vi "frontend.vi"() -> ()   [LabVIEW 2011]
uses:
  custom_modules/typedefs/point.ctl
  custom_modules/typedefs/control_cluster.ctl
  custom_modules/typedefs/preset_control_cluster.ctl
  custom_modules/typedefs/single_step_controls.ctl
  custom_modules/typedefs/camera_settings.ctl
  labview tests/states.ctl
  <vilib>/Utility/error.llb/DialogType.ctl
  stage_modules/Globals.vi
  <vilib>/vision/NI_Vision_Development_Module.lvlib
panel:
  in  "Single step controls":T1
  in  "emergency stop":bool
  in  "Control tabs":T2(tab)
  in  "File name base":string
  in  "Movement controls":T3={"Nx"=10, "Ny"=10, "X separation"=100, "Y separation"=100}
  in  "set origin button":bool
  in  "Preset controls":T4 {"Presets" items=["test1.preset", "test2.preset"]}
  in  "Origin":T5
  in  "PC connection port":u16(ring)=3 items=["PCI board", "COM 1", "TPL1", "COM3"]
  in  "close button":bool
  in  "Run test button":bool
  in  "params_changed":bool
  out "connection indicator":bool
  in  "stage adjusted":bool
  out "Most recent image":T6(plugin-control)
  out "Image index":i32
  out "Preview":T6(plugin-control)
  out "Histogram":T7(graph)
  in  "Camera settings":T8={"Gain"=1.0, "Exposure (s)"=0.05, "Preview binning"=2, "Capture binning"=0} {"Capture binning" items=["1x1", "2x2", "4x4", "8x8"]; "Preview binning" items=["1x1", "2x2", "4x4", "8x8"]; "Exposure (s)" scale=1e-05..1000.0 scale format="%^#_1e"; "Gain" scale=0.451..21.5 scale format="%#_3g"}
  in  "auto expose button":bool
  in  "Delay between captures (ms)":dbl=2000.0
  in  "Image Output directory":path=path "C:/Users/0800706m/Documents/microscope_software/output"
  in  "Preset directory":path=path "C:/Users/0800706m/Documents/microscope_software/presets"
  in  "Focal stack separation":dbl
  in  "Focal stack size":i32
  out "Array of positions":T5[](array[typedef])
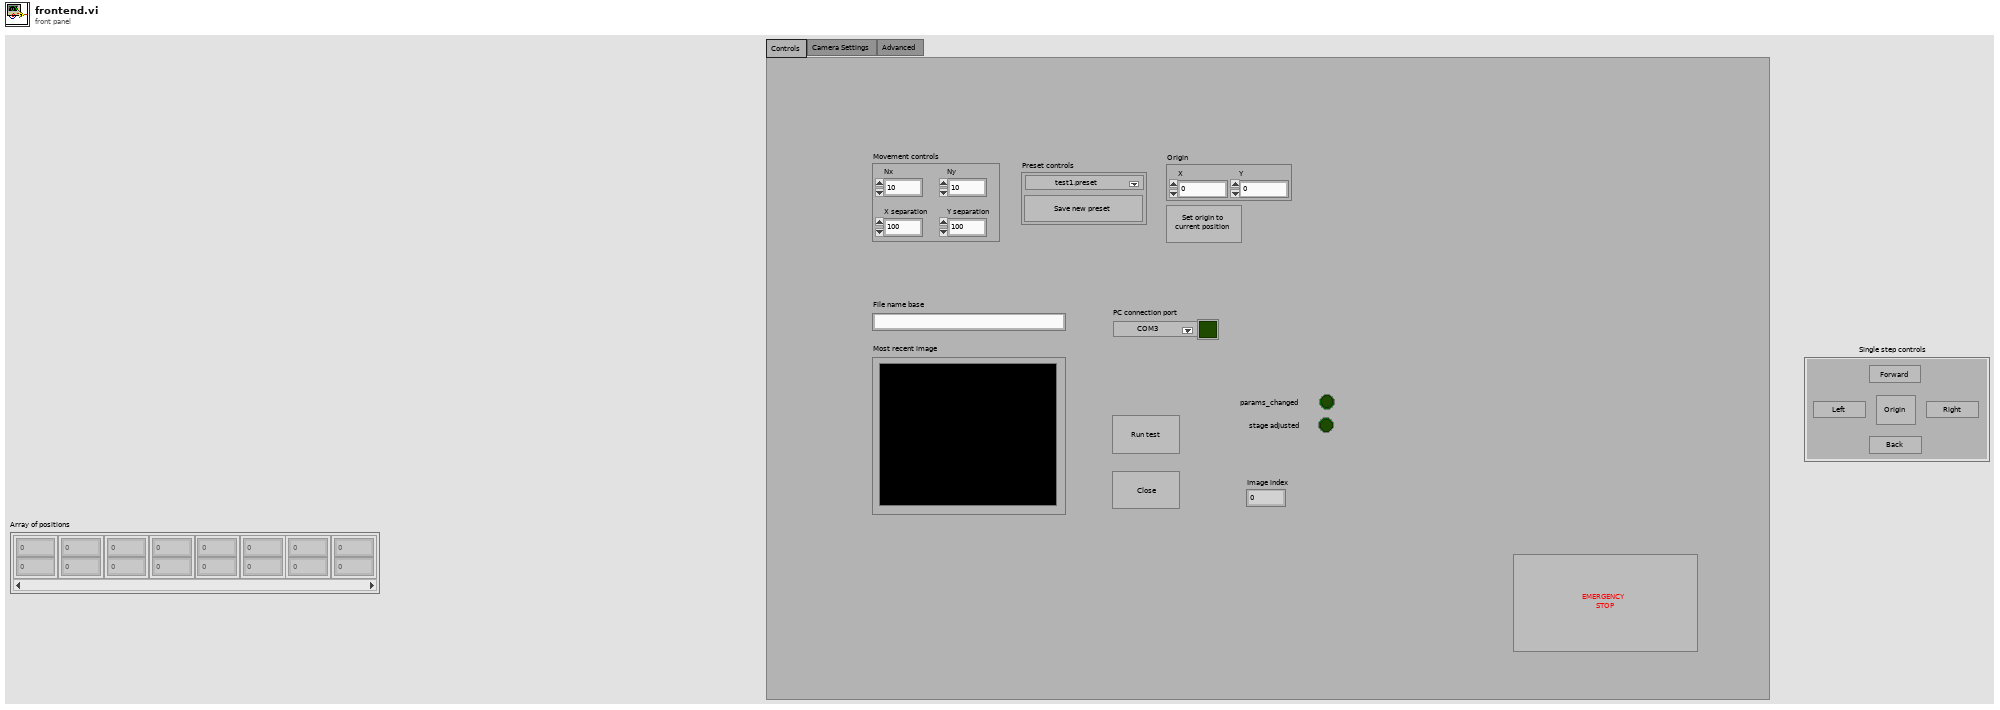
[diagram p1: front panel]
types:
  T1 = typedef "single_step_controls.ctl" = cluster{"move to origin button":bool, "Left":bool, "Right":bool, "Back":bool, "Forward":bool}
  T2 = enum32{"Controls", "Camera Settings", "Advanced"}
  T3 = typedef "control_cluster.ctl" = cluster{"Nx":i32, "Ny":i32, "X separation":i32, "Y separation":i32}
  T4 = typedef "preset_control_cluster.ctl" = cluster{"Presets":u16, "save preset button":bool}
  T5 = typedef "point.ctl" = cluster{"X":i32, "Y":i32}
  T6 = typedef "IMAQ Image.ctl" = refnum<image>
  T7 = cluster{"Starting Value":sgl, "Incremental Value":sgl, "Histogram":u32[]}
  T8 = typedef "camera_settings.ctl" = cluster{"Gain":dbl, "Exposure (s)":dbl, "Preview binning":u16, "Capture binning":u16}
  T9 = typedef "states.ctl" = enum16{"Init", "Check state", "Set parameters", "Preview", "Adjust stage", "Run test", "Close"}
  T10 = enum8{"Enabled", "Disabled", "Disabled and Grayed Out"}
  T11 = enum32{"gain", "offset", "exposure", "binning", "horizontal binning", "vertical binning", "readout speed", "trigger type", "lcd filter", "cooler", "exposure red", "exposure blue", "image format", "roi x", "roi y", "roi width", "roi height", "reserved1", "shutter state", "reserved2", "sync-b out", "reserved3", "intensifier gain", "trigger delay", "camera mode", "normalized gain", "normalized intenifier gain DB", "doPostProcessing", "postProcessGainRed", "postProcessGainGreen", "postProcessGainBlue", "postProcessBayerAlgorithm", "postProcessImageFormat", "fan", "blackout mode", "high sensitivity", "Readout Port", "EM Gain", "open delay", "close delay", "clearing mode"}
  T12 = typedef "Image Type" = u32
  T13 = cluster{"Refnum out":T6, "cameraId out":u32, "error out":errorcluster}
  T14 = cluster{"Global Rectangle":i32[], "Contours":cluster{"Contour Type":u32, "ROI Type":u32, "Points":i32[]}[]}
  T15 = cluster{"cameraId out":u32, "error out":errorcluster, "Image Out":T6}
  T16 = typedef "DialogType.ctl" = u16
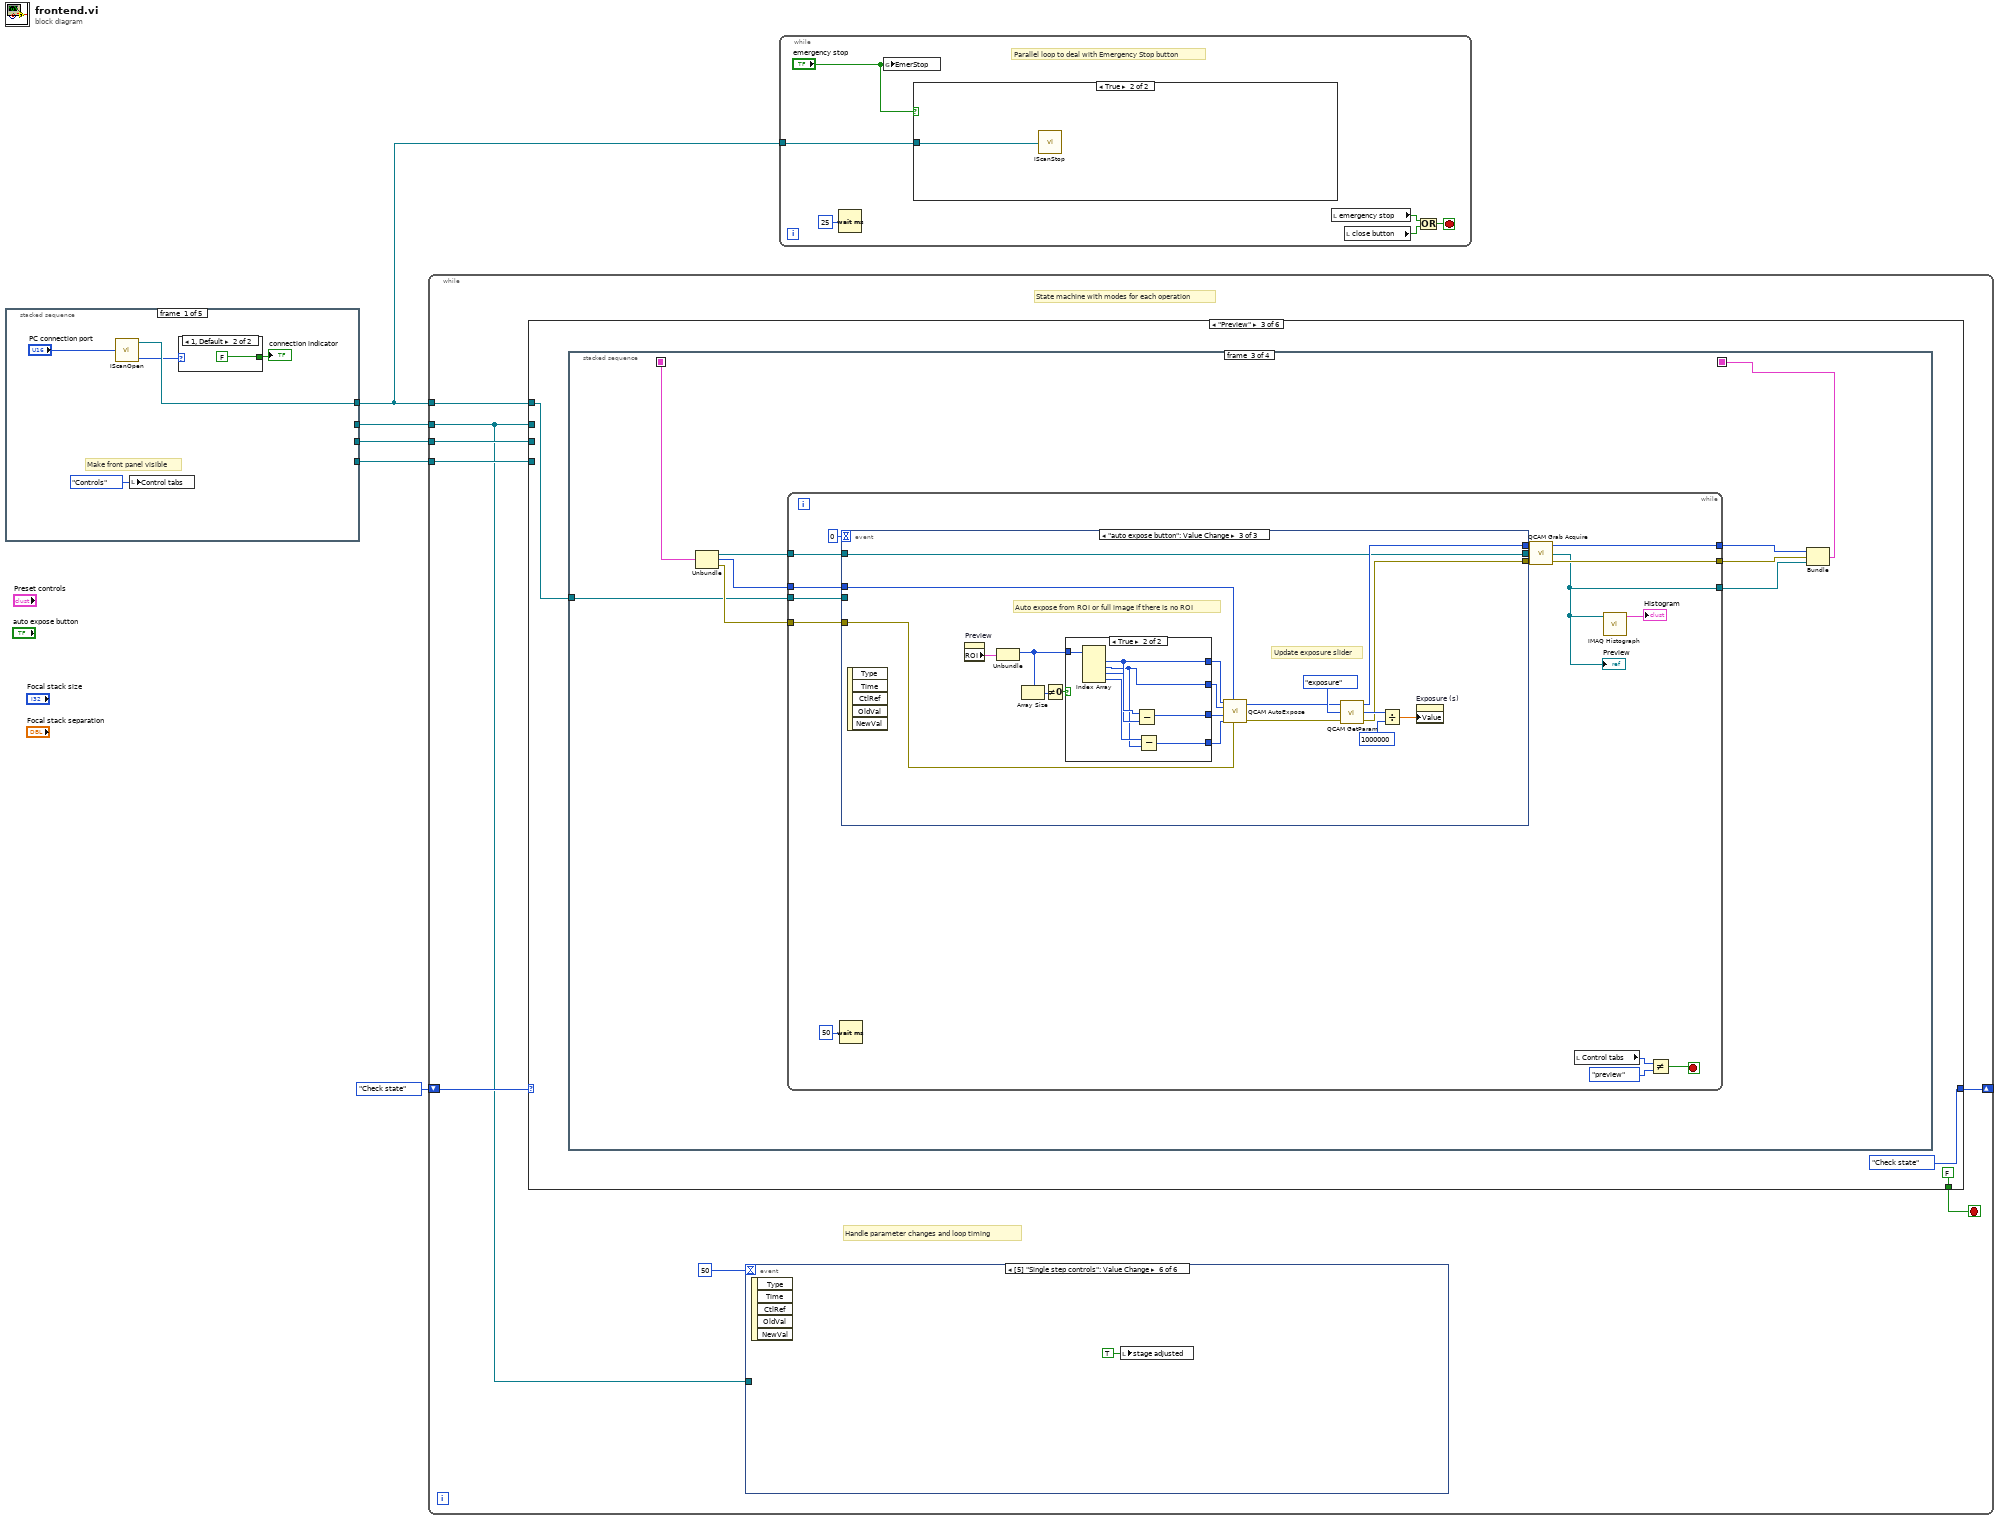
[diagram p0: block diagram]
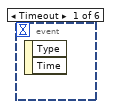
[diagram p3: hidden frame]
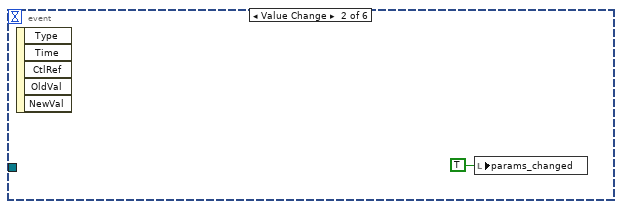
[diagram p4: hidden frame]
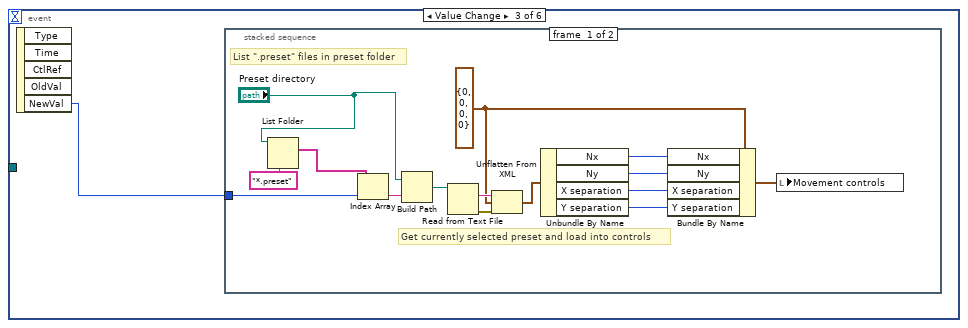
[diagram p5: hidden frame]
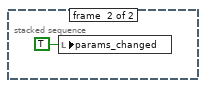
[diagram p6: hidden frame]
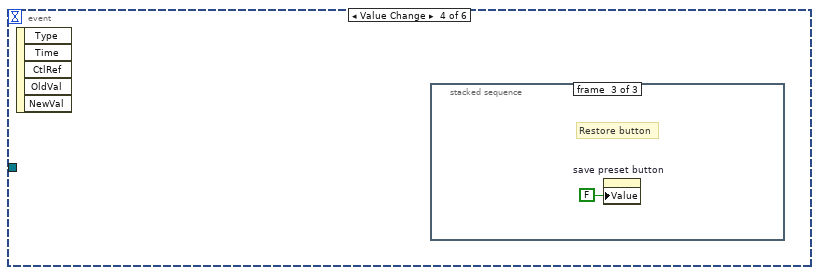
[diagram p7: hidden frame]
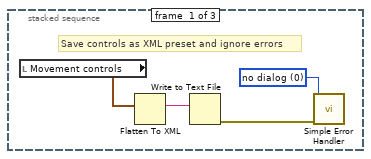
[diagram p8: hidden frame]
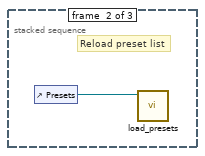
[diagram p9: hidden frame]
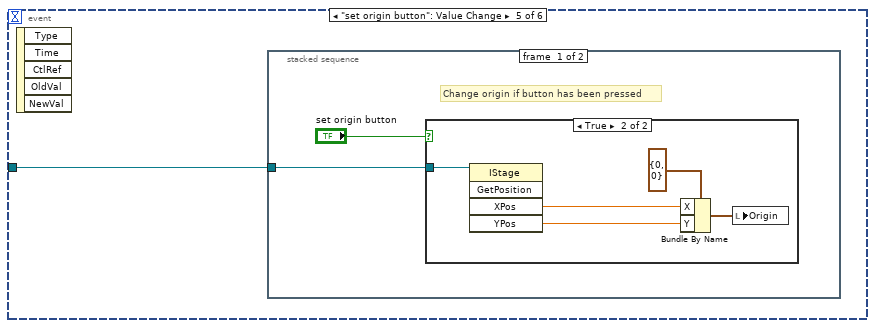
[diagram p10: hidden frame]
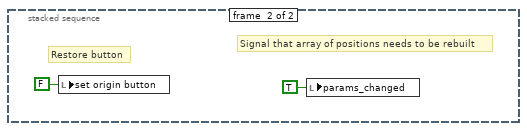
[diagram p12: hidden frame]
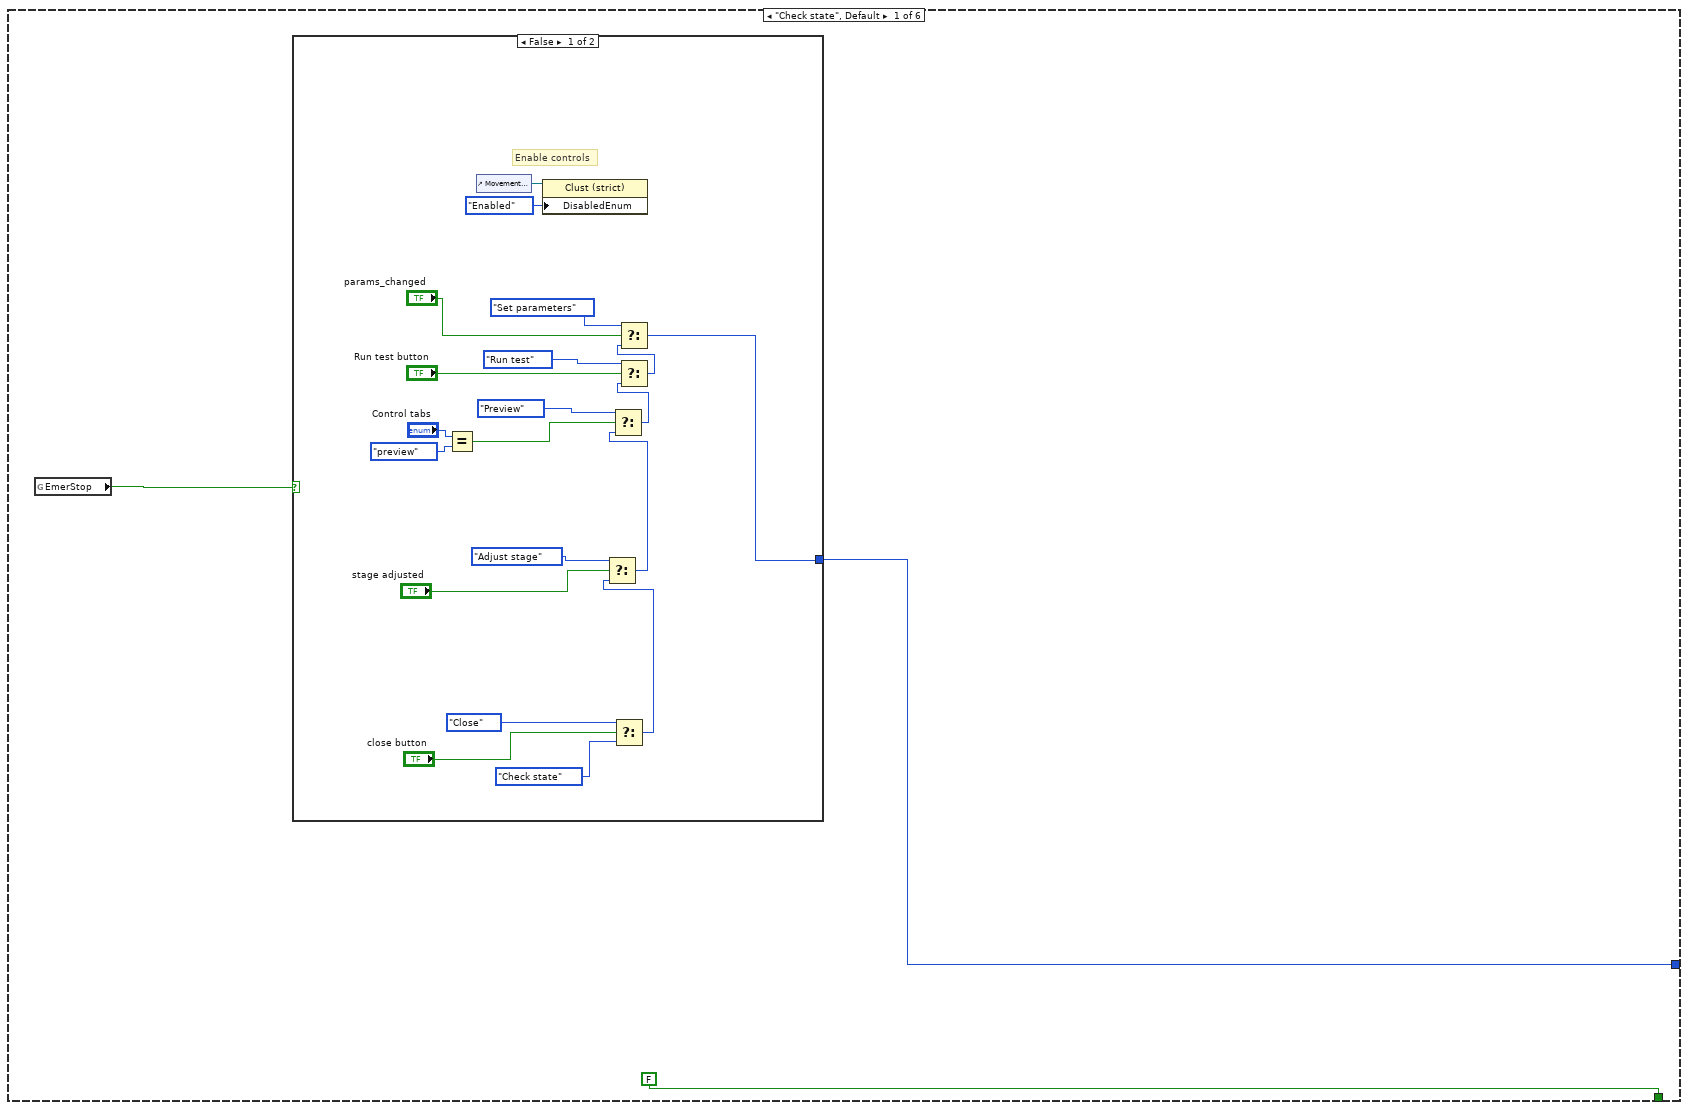
[diagram p13: hidden frame]
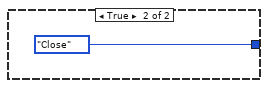
[diagram p14: hidden frame]
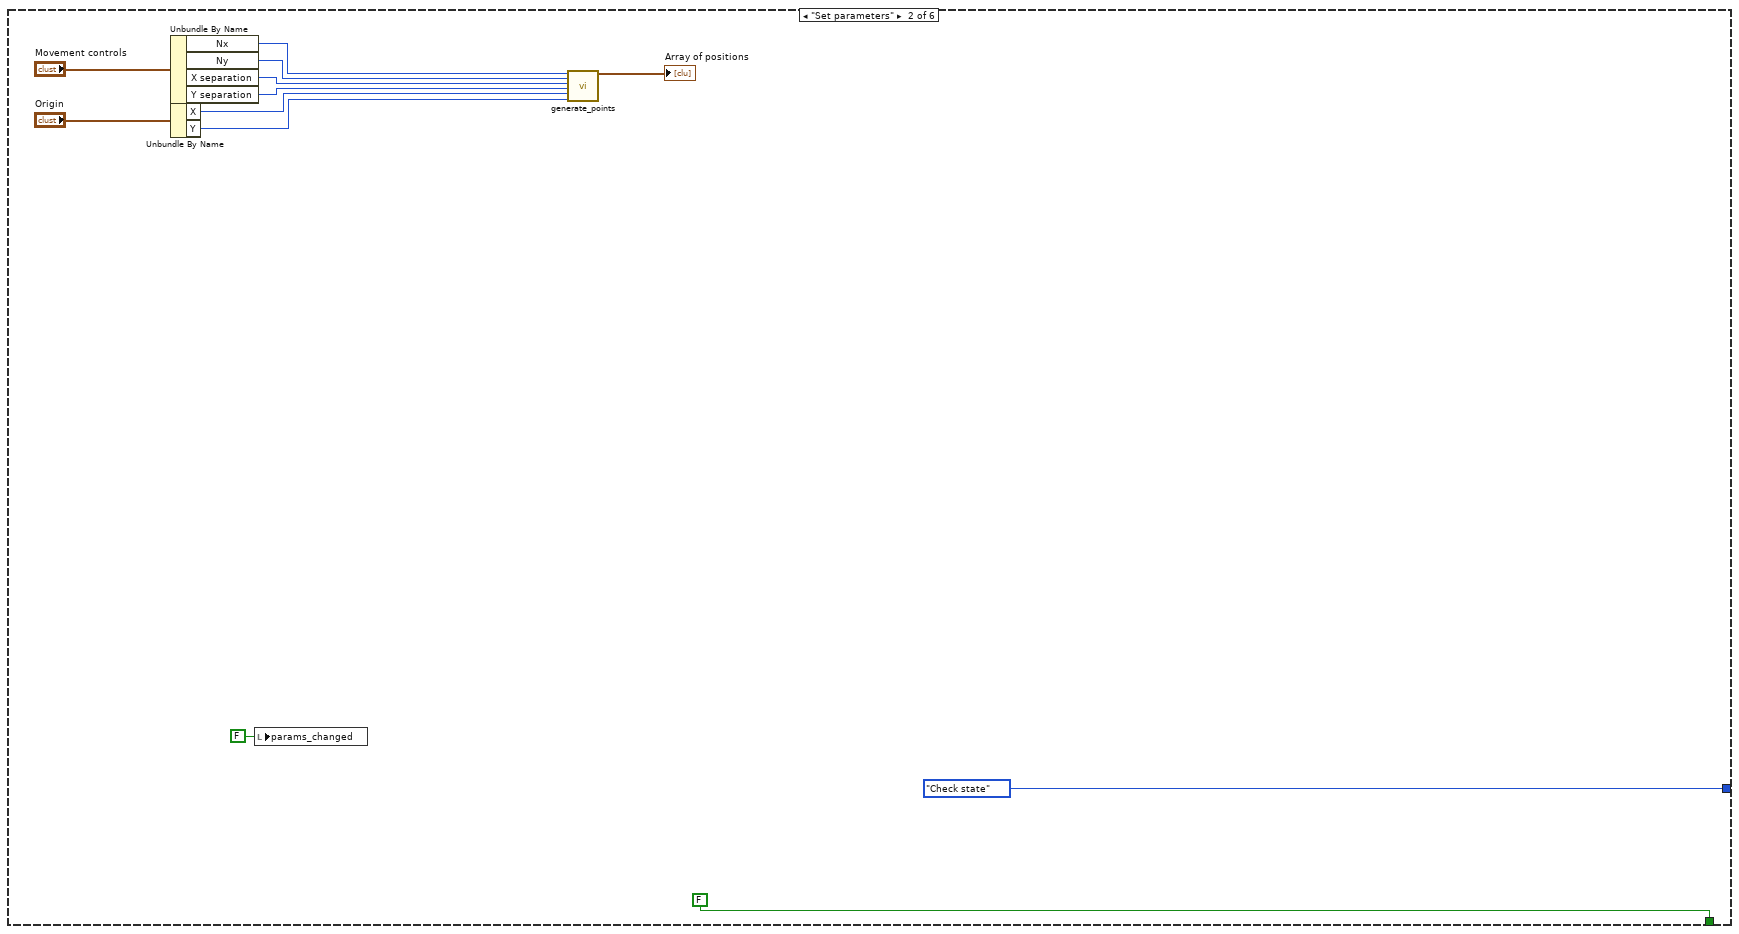
[diagram p15: hidden frame]
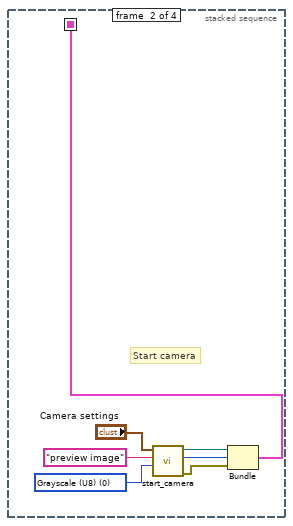
[diagram p17: hidden frame]
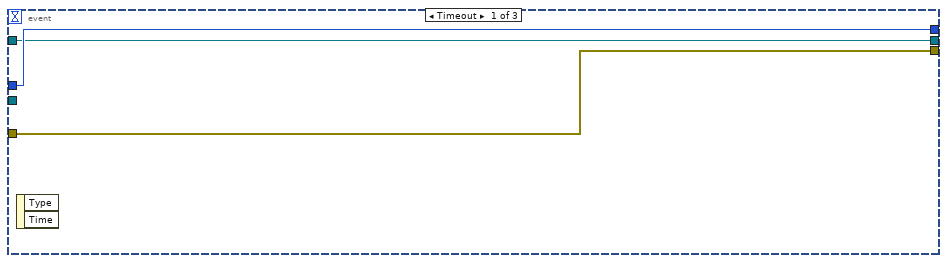
[diagram p18: hidden frame]
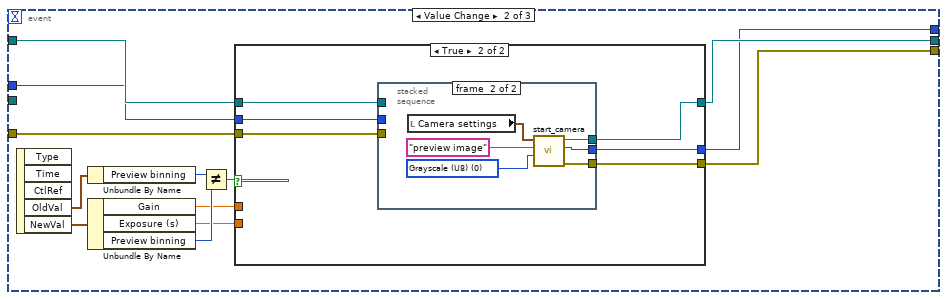
[diagram p19: hidden frame]
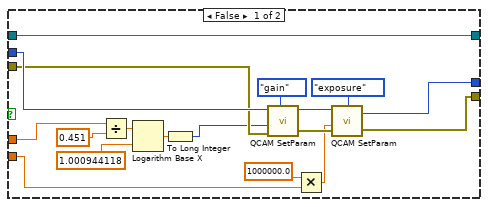
[diagram p20: hidden frame]
diagram:
  n1 = stacked-sequence {
    tunnel: [w10 _ _ _ _] -> w2
    tunnel: [_ w13 _ _ _] -> w1
    tunnel: [_ _ w14 _ _] -> w4
    tunnel: [_ _ _ w15 _] -> w3
    frame #0 {
      # "Make front panel visible"
      n2 = call "IScanOpen.vi"("Port"="PC connection port") -> ("PRIORLib.IScanOut"=w10:refnum<k7>, "Return"=w8:i32)  [unwired: 1 out]
      n3 = local write "Control tabs"(T2."Controls" ("Control tabs")) -> ()
      n4 = case shown="1, Default" w8 {
        tunnel: [TRUE ("connection indicator") FALSE ("connection indicator")] -> w7
        frame 0 {
        }
        frame 1, Default {
        }
      }
      "connection indicator" <- w7
    }
    frame #1 {
      n5 = call "IStageOpen.vi"() -> ("PRIORLib.IStageOut"=w13:refnum<k7>)  [unwired: 1 in, 1 out]
    }
    frame #2 {
      n6 = call "IFilterOpen.vi"() -> ("PRIORLib.IFilterOut"=w14:refnum<k7>)  [unwired: 1 in, 1 out]
    }
    frame #3 {
      n7 = call "IZOpen.vi"() -> ("PRIORLib.IZOut"=w15:refnum<k7>)  [unwired: 1 in, 1 out]
    }
    frame #4 {
      # "Load presets"
      n8 = control-ref of="Presets"() -> (w16:refnum<vi>)
      n9 = call "load_presets.vi"("Ring in"=w16) -> ()  [unwired: 11 in]
    }
  }
  n10 = while {
    shift-right: [w22] -> _
    shift-left: states."Check state" -> [w23]
    tunnel: w2 -> [w18]
    tunnel: w1 -> [w17]
    tunnel: w4 -> [w21]
    tunnel: w3 -> [w20]
    stop <- w24 stop-if-true
    # "Handle parameter changes and loop timing"
    # "State machine with modes for each operation"
    n11 = case shown="\"Preview\"" w23 {
      tunnel: [w60 states."Check state" states."Check state" states."Check state" states."Check state" states."Close"] -> w22
      tunnel: [FALSE FALSE FALSE FALSE FALSE TRUE] -> w24
      tunnel: w18 -> [_ _ w96 w221 w263 w343]
      tunnel: w17 -> [_ _ _ _ _ w342]
      tunnel: w21 -> [_ _ _ _ _ w341]
      tunnel: w20 -> [_ _ _ _ _ w340]
      frame "Check state", Default {
        n12 = global read "Globals.vi" "EmerStop"() -> (w61:bool)
        n13 = case shown="False" w61 {
          tunnel: [w74 states."Close"] -> w60
          frame False {
            # "Enable controls"
            n14 = Equal?(x="Control tabs", y=enum32{"frontend", "preview"}."preview" ("Control tabs")) -> (x = y?=w63:bool)
            n15 = control-ref of="Movement controls"() -> (w72:refnum<vi>)
            n16 = property class="Clust (strict)"(reference=w72, "DisabledEnum"=T10."Enabled" ("Disabled")) -> ()  [unwired: 1 in, 2 out]
            n17 = Select(t=states."Close", s="close button", f=states."Check state") -> (s? t:f=w67:T9)
            n18 = Select(t=states."Adjust stage", s="stage adjusted", f=w67) -> (s? t:f=w68:T9)
            n19 = Select(t=states."Preview", s=w63, f=w68) -> (s? t:f=w70:T9)
            n20 = Select(t=states."Run test", s="Run test button", f=w70) -> (s? t:f=w81:T9)
            n21 = Select(t=states."Set parameters", s="params_changed", f=w81) -> (s? t:f=w74:T9)
          }
          frame True {
          }
        }
      }
      frame "Set parameters" {
        n22 = Unbundle By Name("Movement controls") -> ("Nx"=w87:i32, "Ny"=w88:i32, "X separation"=w89:i32, "Y separation"=w90:i32)
        n23 = Unbundle By Name("Origin") -> ("X"=w84:i32, "Y"=w85:i32)
        n24 = local write "params_changed"(FALSE ("params_changed")) -> ()
        n25 = call "generate_points.vi"("nx"=w87, "ny"=w88, "sepx"=w89, "sepy"=w90, "offsetx"=w84, "offsety"=w85) -> ("Array of positions"=→"Array of positions":T5[])  [unwired: 13 in]
      }
      frame "Preview" {
        n26 = stacked-sequence {
          seq-local: [_ w99 _ _] -> [_ _ w114 _]
          seq-local: [_ _ w107 _] -> [_ _ _ w214]
          tunnel: w96 -> [_ _ w106 _]
          frame #0 {
          }
          frame #1 {
            w105 = T12 0 items=["Grayscale (U8)", "Grayscale (I16)", "Grayscale (SGL)", "Complex (CSG)", "RGB (U32)", "HSL (U32)", "RGB (U64)"] ("Image Type")
            # "Start camera"
            n27 = call "start_camera.vi"("Image Type"=w105, "String"="preview image", "Camera settings"="Camera settings") -> ("error out"=w100:errorcluster, "cameraId out"=w101:u32, "Refnum out"=w102:T6)  [unwired: 6 in]
            n28 = Bundle("Refnum out"=w102, "cameraId out"=w101, "error out"=w100) -> (w99:T13)  [unwired: 1 in]
          }
          frame #2 {
            n29 = Unbundle(w114) -> ("Refnum out"=w113:T6, "cameraId out"=w112:u32, "error out"=w111:errorcluster)
            n30 = while {
              tunnel: w112 -> [w123]
              tunnel: w111 -> [w124]
              tunnel: w113 -> [w119]
              tunnel: [w130] -> w110
              tunnel: [w129] -> w109
              tunnel: [w125] -> w108
              tunnel: w106 -> [w115]
              stop <- w118 stop-if-true
              n31 = Wait (ms)(milliseconds to wait=u32 50) -> ()  [unwired: 1 out]
              n32 = event shown="[2] \"auto expose button\": Value Change" {
                selector: _ -> [_ _ _]
                dyn-events: _ -> [_ _ _]
                timeout: 0 -> [_ _ _]
                tunnel: w124 -> [w131 w138 w183]
                tunnel: w123 -> [w133 w137 w188]
                tunnel: [w133 w135 w186] -> w122
                tunnel: [w132 w136 w182] -> w121
                tunnel: [w131 w134 w185] -> w120
                tunnel: w119 -> [w132 w141 w182]
                tunnel: w115 -> [_ _ _]
                event Timeout {
                  n33 = event-data() -> ()  [unwired: 1 in, 2 out]
                }
                event Value Change {
                  n34 = event-data() -> ("OldVal"=w145:T8, "NewVal"=w146:T8)  [unwired: 1 in, 3 out]
                  n35 = Unbundle By Name(w145) -> ("Preview binning"=w144:u16)
                  n36 = Unbundle By Name(w146) -> ("Gain"=w140:dbl, "Exposure (s)"=w139:dbl, "Preview binning"=w142:u16)
                  n37 = Not Equal?(x=w142, y=w144) -> (x != y?=w143:bool)
                  n38 = case shown="True" w143 {
                    tunnel: w138 -> [w153 w170]
                    tunnel: w141 -> [w164 w169]
                    tunnel: [w164 w168] -> w136
                    tunnel: w140 -> [w147 _]
                    tunnel: w139 -> [w157 _]
                    tunnel: w137 -> [w156 w167]
                    tunnel: [w155 w166] -> w135
                    tunnel: [w154 w165] -> w134
                    frame False {
                      n39 = Divide(x=w147, y=0.451) -> (x/y=w151:dbl)
                      n40 = Logarithm Base X(1:1.000944118 ("x"), 2:w151) -> (0:w149:dbl)
                      n41 = To Long Integer(number=w149) -> (32bit integer=w148:i32)
                      n42 = call <userlib>:"QCAM SetParam.vi"("error in (no error)"=w153, "value"=w148, "parameter key"=T11."gain", "cameraId"=w156) -> ("error out"=w162:errorcluster, "cameraId out"=w161:u32)
                      n43 = Multiply(x=1000000.0, y=w157) -> (x*y=w160:dbl)
                      n44 = call <userlib>:"QCAM SetParam.vi"("error in (no error)"=w162, "value"=w160, "parameter key"=T11."exposure", "cameraId"=w161) -> ("error out"=w154:errorcluster, "cameraId out"=w155:u32)
                    }
                    frame True {
                      n45 = stacked-sequence {
                        tunnel: w170 -> [w172 _]
                        tunnel: w169 -> [_ _]
                        tunnel: [_ w177] -> w168
                        tunnel: w167 -> [w171 _]
                        tunnel: [_ w176] -> w166
                        tunnel: [_ w175] -> w165
                        frame #0 {
                          n46 = call <userlib>:"QCAM Grab Stop.vi"("error in (no error)"=w172, "cameraId"=w171) -> ("error out"=w173:errorcluster, "cameraId Out"=w174:u32)
                          n47 = call <userlib>:"QCAM Close.vi"("error in (no error)"=w173, "cameraId"=w174) -> ()  [unwired: 1 in, 1 out]
                        }
                        frame #1 {
                          w180 = T12 0 items=["Grayscale (U8)", "Grayscale (I16)", "Grayscale (SGL)", "Complex (CSG)", "RGB (U32)", "HSL (U32)", "RGB (U64)"] ("Image Type")
                          n48 = local read "Camera settings"() -> (w178:T8)
                          n49 = call "start_camera.vi"("Image Type"=w180, "String"="preview image", "Camera settings"=w178) -> ("error out"=w175:errorcluster, "cameraId out"=w176:u32, "Refnum out"=w177:T6)  [unwired: 6 in]
                        }
                      }
                    }
                  }
                }
                event "auto expose button": Value Change {
                  # "Auto expose from ROI or full image if there is no ROI"
                  # "Update exposure slider"
                  n50 = event-data() -> ()  [unwired: 1 in, 5 out]
                  n51 = property on="Preview" class="ImageControl"() -> ("ROI"=w189:T14)  [unwired: 2 in, 2 out]
                  n52 = Unbundle(w189) -> ("Global Rectangle"=w190:i32[])  [unwired: 1 out]
                  n53 = Array Size(array=w190) -> (size(s)=w191:i32)
                  n54 = Not Equal To 0?(x=w191) -> (x != 0?=w192:bool)
                  n55 = case shown="True" w192 {
                    tunnel: w190 -> [_ w208]
                    tunnel: [w200 w207] -> w193
                    tunnel: [w200 w206] -> w194
                    tunnel: [w201 w205] -> w195
                    tunnel: [w202 w204] -> w196
                    frame False {
                      w200 = 0
                      n56 = local read "Preview"() -> (w203:T6)
                      n57 = call "IMAQ GetImageSize"("Image"=w203) -> ("Y Resolution"=w202:i32, "X Resolution"=w201:i32)  [unwired: 3 in, 1 out]
                    }
                    frame True {
                      n58 = Index Array(array=w208) -> (element #1=w207:i32, element #2=w206:i32, element #3=w210:i32, element #4=w209:i32)  [unwired: 4 in]
                      n59 = Subtract(x=w210, y=w207) -> (x-y=w205:i32)
                      n60 = Subtract(x=w209, y=w206) -> (x-y=w204:i32)
                    }
                  }
                  n61 = call <userlib>:"QCAM AutoExpose.vi"("xOrig"=w193, "cameraId"=w188, "yOrig"=w194, "width"=w195, "error in (no error)"=w183, "height"=w196) -> ("cameraId out"=w187:u32, "error out"=w184:errorcluster)  [unwired: 1 in]
                  n62 = call <userlib>:"QCAM GetParam.vi"("cameraId in"=w187, "parameter key"=T11."exposure", "error in (no error)"=w184) -> ("cameraId out"=w186:u32, "value out"=w197:u32, "error out"=w185:errorcluster)  [unwired: 2 out]
                  n63 = Divide(x=w197, y=1000000) -> (x/y=w181:dbl)
                  n64 = property on="Exposure (s)" class="Slide (strict)"("Value"=w181) -> ()  [unwired: 2 in, 2 out]
                }
              }
              n65 = call <userlib>:"QCAM Grab Acquire.vi"("error in (no error)"=w120, "Image"=w121, "cameraId"=w122) -> ("error out"=w129:errorcluster, "Image Out"=w125:T6, "cameraId out"=w130:u32)
              "Preview" <- w125
              n66 = local read "Control tabs"() -> (w117:T2)
              n67 = call "IMAQ Histograph"("Image"=w125) -> ("Histogram Graph"=→"Histogram":T7)  [unwired: 7 in, 3 out]
              n68 = Not Equal?(x=w117, y=enum32{"frontend", "preview"}."preview" ("Control tabs")) -> (x != y?=w118:bool)
            }
            n69 = Bundle("cameraId out"=w110, "error out"=w109, "Image Out"=w108) -> (w107:T15)  [unwired: 1 in]
          }
          frame #3 {
            # "Close everything"
            n70 = Unbundle(w214) -> ("cameraId out"=w213:u32, "error out"=w212:errorcluster, "Image Out"=w211:T6)
            n71 = call <userlib>:"QCAM Grab Stop.vi"("error in (no error)"=w212, "cameraId"=w213) -> ("error out"=w215:errorcluster, "cameraId Out"=w216:u32)
            n72 = call "IMAQ Dispose"("Image"=w211) -> ()  [unwired: 5 in, 1 out]
            n73 = call <userlib>:"QCAM Close.vi"("error in (no error)"=w215, "cameraId"=w216) -> ()  [unwired: 1 in, 1 out]
          }
        }
      }
      frame "Adjust stage" {
        # "Cycle through buttons and execute the one that has been pressed"
        n74 = local read "Movement controls"() -> (w219:T3)
        n75 = Unbundle By Name(w219) -> ("X separation"=w217:i32, "Y separation"=w218:i32)
        n76 = stacked-sequence {
          tunnel: w221 -> [w226 w232 w240 w247 w255 _]
          tunnel: "Single step controls" -> [w224 w235 w243 w250 w258 _]
          tunnel: w218 -> [_ _ _ w248 w256 _]
          tunnel: w217 -> [_ w233 w241 _ _ _]
          frame #0 {
            n77 = Unbundle By Name(w224) -> ("move to origin button"=w225:bool)
            n78 = case shown="True" w225 {
              tunnel: w226 -> [_ w227]
              frame False {
              }
              frame True {
                n79 = local read "Origin"() -> (w231:T5)
                n80 = Unbundle By Name(w231) -> ("X"=w229:i32, "Y"=w228:i32)
                n81 = call "IScanMoveXYZAbs.vi"("ZPos"=0.0, "YPos"=w228, "XPos"=w229, "PRIORLib.IScanIn"=w227) -> ()  [unwired: 3 out]
              }
            }
          }
          frame #1 {
            n82 = Unbundle By Name(w235) -> ("Left"=w234:bool)
            n83 = case shown="True" w234 {
              tunnel: w233 -> [_ w239]
              tunnel: w232 -> [_ w236]
              frame False {
              }
              frame True {
                w237 = 0.0 ("ZPos")
                n84 = Negate(x=w239) -> (-x=w238:i32)
                n85 = call "IScanMoveXYZ.vi"("ZPos"=w237, "YPos"=w237, "XPos"=w238, "PRIORLib.IScanIn"=w236) -> ()  [unwired: 3 out]
              }
            }
          }
          frame #2 {
            n86 = Unbundle By Name(w243) -> ("Right"=w242:bool)
            n87 = case shown="True" w242 {
              tunnel: w241 -> [_ w245]
              tunnel: w240 -> [_ w244]
              frame False {
              }
              frame True {
                w246 = 0.0 ("ZPos")
                n88 = call "IScanMoveXYZ.vi"("ZPos"=w246, "YPos"=w246, "XPos"=w245, "PRIORLib.IScanIn"=w244) -> ()  [unwired: 3 out]
              }
            }
          }
          frame #3 {
            n89 = Unbundle By Name(w250) -> ("Back"=w249:bool)
            n90 = case shown="True" w249 {
              tunnel: w248 -> [_ w254]
              tunnel: w247 -> [_ w251]
              frame False {
              }
              frame True {
                w252 = 0.0 ("ZPos")
                n91 = Negate(x=w254) -> (-x=w253:i32)
                n92 = call "IScanMoveXYZ.vi"("ZPos"=w252, "YPos"=w253, "XPos"=w252, "PRIORLib.IScanIn"=w251) -> ()  [unwired: 3 out]
              }
            }
          }
          frame #4 {
            n93 = Unbundle By Name(w258) -> ("Forward"=w257:bool)
            n94 = case shown="True" w257 {
              tunnel: w256 -> [_ w261]
              tunnel: w255 -> [_ w259]
              frame False {
              }
              frame True {
                w260 = 0.0 ("ZPos")
                n95 = call "IScanMoveXYZ.vi"("ZPos"=w260, "YPos"=w261, "XPos"=w260, "PRIORLib.IScanIn"=w259) -> ()  [unwired: 3 out]
              }
            }
          }
          frame #5 {
            n96 = local write "stage adjusted"(FALSE ("stage adjusted")) -> ()
          }
        }
      }
      frame "Run test" {
        n97 = stacked-sequence {
          seq-local: [w266 _ _] -> [_ w278 w334]
          tunnel: w263 -> [_ w279 _]
          frame #0 {
            w272 = T12 0 items=["Grayscale (U8)", "Grayscale (I16)", "Grayscale (SGL)", "Complex (CSG)", "RGB (U32)", "HSL (U32)", "RGB (U64)"] ("Image Type")
            # "Start camera"
            # "Disable controls during test"
            n98 = local read "Camera settings"() -> (w267:T8)
            n99 = control-ref of="Movement controls"() -> (w273:refnum<vi>)
            n100 = property class="Clust (strict)"(reference=w273, "DisabledEnum"=T10."Disabled and Grayed Out" ("Disabled")) -> ()  [unwired: 1 in, 2 out]
            n101 = call "start_camera.vi"("Image Type"=w272, "String"="capture image", "Camera settings"=w267) -> ("error out"=w268:errorcluster, "cameraId out"=w269:u32, "Refnum out"=w270:T6)  [unwired: 6 in]
            n102 = Bundle("Refnum out"=w270, "cameraId out"=w269, "error out"=w268) -> (w266:T13)  [unwired: 1 in]
          }
          frame #1 {
            n103 = Unbundle(w278) -> ("Refnum out"=w276:T6, "cameraId out"=w277:u32)  [unwired: 1 out]
            n104 = local read "Movement controls"() -> (w280:T3)
            n105 = Unbundle By Name(w280) -> ("Nx"=w281:i32, "Ny"=w275:i32)
            n106 = for {
              N: w281 -> [w283]
              tunnel: w279 -> [w288]
              tunnel: w277 -> [w286]
              tunnel: w276 -> [w285]
              tunnel: w275 -> [w284]
              i -> [w296]
              stop <- w287 stop-if-true
              # "Reverse every other row"
              n107 = Multiply(x=w296, y=w283) -> (x*y=w282:i32)
              n108 = local read "Array of positions"() -> (w297:T5[])
              n109 = Quotient & Remainder(x=w296, y=2) -> (x-y*floor(x/y)=w294:i32)  [unwired: 1 out]
              n110 = Equal?(x=w294, y=0) -> (x = y?=w292:bool)
              n111 = Array Subset(array=w297, index=w282, length=w283) -> (w290:T5[])
              n112 = Reverse 1D Array(array=w290) -> (reversed array=w291:T5[])
              n113 = Select(t=w290, s=w292, f=w291) -> (s? t:f=w289:T5[])
              n114 = for {
                N: w284 -> [_]
                tunnel: w289 -> [w304] mode=indexing
                tunnel: w288 -> [w305]
                tunnel: w286 -> [w302]
                tunnel: w285 -> [w301]
                tunnel: w282 -> [w299]
                i -> [w300]
                stop <- w303 stop-if-true
                n115 = Add(x=w299, y=w300) -> (x+y=→"Image index":i32)
                n116 = stacked-sequence {
                  tunnel: w305 -> [_ w309 w315 _ _]
                  tunnel: w304 -> [_ w308 _ _ _]
                  tunnel: w302 -> [_ _ _ w329 _]
                  tunnel: w301 -> [_ _ _ w328 _]
                  frame #0 {
                    # "Delay to stop movement blur"
                    n117 = Wait (ms)(milliseconds to wait="Delay between captures (ms)") -> ()  [unwired: 1 out]
                  }
                  frame #1 {
                    n118 = global read "Globals.vi" "EmerStop"() -> (w307:bool)
                    n119 = case shown="False" w307 {
                      tunnel: w309 -> [w314 _]
                      tunnel: w308 -> [w313 _]
                      frame False {
                        n120 = Unbundle(w313) -> ("X"=w311:i32, "Y"=w310:i32)
                        n121 = call "IScanMoveXYZAbs.vi"("ZPos"=0.0, "YPos"=w310, "XPos"=w311, "PRIORLib.IScanIn"=w314) -> ()  [unwired: 3 out]
                      }
                      frame True {
                      }
                    }
                  }
                  frame #2 {
                    n122 = while {
                      tunnel: w315 -> [w321]
                      stop <- w317 continue-if-true
                      # "Wait until stage has moved."
                      n123 = invoke class="IScan" method="IsMoving"(reference=w321) -> ("Status"=w316:i32)  [unwired: 3 in, 3 out]
                      n124 = global read "Globals.vi" "EmerStop"() -> (w319:bool)
                      n125 = Not(x=w319) -> (.not. x?=w318:bool)
                      n126 = Greater Than 0?(x=w316) -> (x > 0?=w320:bool)
                      n127 = And(x=w320, y=w318) -> (x .and. y?=w317:bool)
                    }
                  }
                  frame #3 {
                    n128 = local read "Image index"() -> (w327:i32)
                    n129 = call <userlib>:"QCAM Grab Acquire.vi"("Image"=w328, "cameraId"=w329) -> ("Image Out"=w325:T6)  [unwired: 1 in, 2 out]
                    "Most recent image" <- w325
                    n130 = call "Build Text"("Beginning Text"="File name base", "index"=w327) -> ("Result"=w323:string)  [unwired: 12 in, 1 out]
                    n131 = Build Path(base path="Image Output directory", name or relative path=w323) -> (appended path=w322:path)
                    n132 = call-poly "IMAQ Write File 2"("File Path"=w322, "Image"=w325) -> ()  [unwired: 8 in, 2 out]
                  }
                  frame #4 {
                    # "Wait until exposure is finshed and increment image number"
                    n133 = local read "Camera settings"() -> (w333:T8)
                    n134 = Unbundle By Name(w333) -> ("Exposure (s)"=w332:dbl)
                    n135 = Multiply(x=1000.0, y=w332) -> (x*y=w330:dbl)
                    n136 = Wait (ms)(milliseconds to wait=w330) -> ()  [unwired: 1 out]
                  }
                }
                n137 = global read "Globals.vi" "EmerStop"() -> (w303:bool)
              }
              n138 = global read "Globals.vi" "EmerStop"() -> (w287:bool)
            }
          }
          frame #2 {
            # "Close everything"
            n139 = Unbundle(w334) -> ("Refnum out"=w335:T6, "cameraId out"=w337:u32, "error out"=w336:errorcluster)
            n140 = call <userlib>:"QCAM Grab Stop.vi"("error in (no error)"=w336, "cameraId"=w337) -> ("error out"=w338:errorcluster, "cameraId Out"=w339:u32)
            n141 = call "IMAQ Dispose"("Image"=w335) -> ()  [unwired: 5 in, 1 out]
            n142 = call <userlib>:"QCAM Close.vi"("error in (no error)"=w338, "cameraId"=w339) -> ()  [unwired: 1 in, 1 out]
          }
        }
      }
      frame "Close" {
        # "Clean up at the end. The last command issued\nis IScan.Disconnect, done whithin IScanClose."
        n143 = stacked-sequence {
          tunnel: w343 -> [_ _ _ w349 _]
          tunnel: w342 -> [_ _ w348 _ _]
          tunnel: w341 -> [w346 _ _ _ _]
          tunnel: w340 -> [_ w347 _ _ _]
          frame #0 {
            n144 = call "IFilterClose.vi"("PRIORLib.IFilter"=w346) -> ()  [unwired: 1 out]
          }
          frame #1 {
            n145 = call "IZClose.vi"("PRIORLib.IZ"=w347) -> ()  [unwired: 1 out]
          }
          frame #2 {
            n146 = call "IStageClose.vi"("PRIORLib.IStage"=w348) -> ()  [unwired: 1 out]
          }
          frame #3 {
            n147 = call "IScanClose.vi"("PRIORLib.IScan"=w349) -> ()  [unwired: 2 out]
          }
          frame #4 {
            w350 = FALSE
            n148 = local write "connection indicator"(w350) -> ()
            n149 = local write "emergency stop"(w350) -> ()
            n150 = local write "close button"(w350) -> ()
          }
        }
      }
    }
    n151 = event shown="[5] \"Single step controls\": Value Change" {
      selector: _ -> [_ _ _ _ _ _]
      dyn-events: _ -> [_ _ _ _ _ _]
      timeout: 50 -> [_ _ _ _ _ _]
      tunnel: w17 -> [_ _ _ _ w49 _]
      event Timeout {
        n152 = event-data() -> ()  [unwired: 1 in, 2 out]
      }
      event Value Change {
        n153 = event-data() -> ()  [unwired: 1 in, 5 out]
        n154 = local write "params_changed"(TRUE ("params_changed")) -> ()
      }
      event Value Change {
        n155 = event-data() -> ("NewVal"=w26:u16)  [unwired: 1 in, 4 out]
        n156 = stacked-sequence {
          tunnel: w26 -> [w28 _]
          frame #0 {
            w37 = T3 {"Nx"=0, "Ny"=0, "X separation"=0, "Y separation"=0} ("controls")
            # "Get currently selected preset and load into controls"
            # "List \".preset\" files in preset folder"
            n157 = List Folder(path="Preset directory", pattern="*.preset") -> (filenames=w30:string[])  [unwired: 2 in, 3 out]
            n158 = Index Array(array=w30, index=w28) -> (element=w29:string)
            n159 = Build Path(base path="Preset directory", name or relative path=w29) -> (appended path=w39:path)
            n160 = Read from Text File(file (use dialog)=w39) -> (text=w41:string, error out=w40:errorcluster)  [unwired: 3 in, 2 out]
            n161 = Unflatten From XML(xml string=w41, type=w37, error in (no error)=w40) -> (value=w38:T3)  [unwired: 1 out]
            n162 = Unbundle By Name(w38) -> ("Nx"=w36:i32, "Ny"=w35:i32, "X separation"=w34:i32, "Y separation"=w33:i32)
            n163 = Bundle By Name(cluster=w37, "Nx"=w36, "Ny"=w35, "X separation"=w34, "Y separation"=w33) -> (w32:T3)
            n164 = local write "Movement controls"(w32) -> ()
          }
          frame #1 {
            n165 = local write "params_changed"(TRUE ("params_changed")) -> ()
          }
        }
      }
      event Value Change {
        n166 = event-data() -> ()  [unwired: 1 in, 5 out]
        n167 = stacked-sequence {
          frame #0 {
            w44 = T16 0 items=["no dialog", "OK message", "continue or stop message", "OK message + warnings", "continue/stop + warnings"] ("type of dialog (OK msg:1)")
            # "Save controls as XML preset and ignore errors"
            n168 = local read "Movement controls"() -> (w43:T3)
            n169 = Flatten To XML(anything=w43) -> (xml string=w46:string)
            n170 = Write to Text File(text=w46) -> (error out=w45:errorcluster)  [unwired: 3 in, 2 out]
            n171 = call <vilib>:"Simple Error Handler.vi"("type of dialog (OK msg:1)"=w44, "error in (no error)"=w45) -> ()  [unwired: 3 in, 5 out]
          }
          frame #1 {
            # "Reload preset list"
            n172 = control-ref of="Presets"() -> (w47:refnum<vi>)
            n173 = call "load_presets.vi"("Ring in"=w47) -> ()  [unwired: 11 in]
          }
          frame #2 {
            # "Restore button"
            n174 = property on="save preset button" class="Bool (strict)"("Value"=FALSE) -> ()  [unwired: 2 in, 2 out]
          }
        }
      }
      event "set origin button": Value Change {
        n175 = event-data() -> ()  [unwired: 1 in, 5 out]
        n176 = stacked-sequence {
          tunnel: w49 -> [w50 _]
          frame #0 {
            # "Change origin if button has been pressed"
            n177 = case shown="True" "set origin button" {
              tunnel: w50 -> [_ w54]
              frame False {
              }
              frame True {
                n178 = invoke class="IStage" method="GetPosition"(reference=w54) -> ("XPos"=w53:dbl, "YPos"=w52:dbl)  [unwired: 4 in, 3 out]
                n179 = Bundle By Name(cluster=T5 {"X"=0, "Y"=0} ("point"), "X"=w53, "Y"=w52) -> (w55:T5)
                n180 = local write "Origin"(w55) -> ()
              }
            }
          }
          frame #1 {
            # "Restore button"
            # "Signal that array of positions needs to be rebuilt"
            n181 = local write "set origin button"(FALSE ("set origin button")) -> ()
            n182 = local write "params_changed"(TRUE ("params_changed")) -> ()
          }
        }
      }
      event Value Change {
        n183 = event-data() -> ()  [unwired: 1 in, 5 out]
        n184 = local write "stage adjusted"(TRUE ("stage adjusted")) -> ()
      }
    }
  }
  n185 = while {
    tunnel: w2 -> [w354]
    stop <- w353 stop-if-true
    # "Parallel loop to deal with Emergency Stop button"
    n186 = Wait (ms)(milliseconds to wait=u32 25) -> ()  [unwired: 1 out]
    n187 = global write "Globals.vi" "EmerStop"("emergency stop") -> ()
    n188 = case shown="True" "emergency stop" {
      tunnel: w354 -> [_ w357]
      frame False {
      }
      frame True {
        n189 = call "IScanStop.vi"("PRIORLib.IScanIn"=w357) -> ()  [unwired: 3 out]
      }
    }
    n190 = local read "emergency stop"() -> (w352:bool)
    n191 = local read "close button"() -> (w351:bool)
    n192 = Or(x=w352, y=w351) -> (x .or. y?=w353:bool)
  }
